vi "Deselect Multiple Objects.vi"   [LabVIEW 2023]
doc: "Demonstrates the use of the RemoveFromSelection method in VI Scripting to deselect certain objects that are currently selected."
panel:
  # "Overview: Demonstrates the use of the RemoveFromSelection method in VI Scripting to deselect certain objects that are currently selected.\nInstructions:\n1. Open the block diagram of Test - Selection List Target.vi.\n2. Select at least three top-level objects.\n3. Run this VI. Two of the objects you selected will be deselected, while the remaining objects are still selected. To see this, click the front panel or block diagram window title bar of the Test - Selection List Target.vi after running this VI to make it the active window."
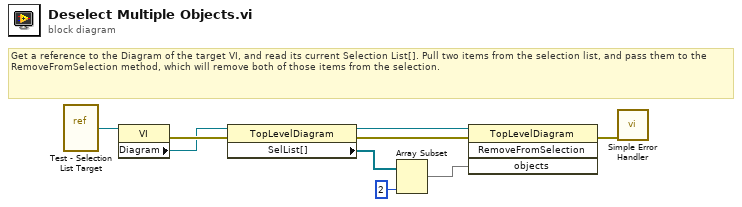
[diagram p0: block diagram]
diagram:
  # "Get a reference to the Diagram of the target VI, and read its current Selection List[]. Pull two items from the selection list, and pass them to the RemoveFromSelection method, which will remove both of those items from the selection."
  n1 = vi-ref "Test - Selection List Target.vi"() -> (w9:refnum<vi>)
  n2 = property class="VI"(reference=w9) -> (error out=w8:errorcluster, "Diagram"=w7:refnum<vi>)  [unwired: 1 in, 1 out]
  n3 = property class="TopLevelDiagram"(reference=w7, error in=w8) -> (reference out=w3:refnum<vi>, error out=w4:errorcluster, "SelList[]"=w6:refnum<vi>[])
  n4 = Array Subset(array=w6, length=2) -> (w2:refnum<vi>[])  [unwired: 1 in]
  n5 = invoke class="TopLevelDiagram" method="RemoveFromSelection"(reference=w3, error in=w4, "objects"=w2) -> (error out=w1:errorcluster)  [unwired: 1 in, 3 out]
  n6 = call <vilib>:"Simple Error Handler.vi"("error in (no error)"=w1) -> ()  [unwired: 4 in, 5 out]
